vi "Manipulator Intake Handler v3.vi"() -> (14 "Manipulator Mode":T1)   [LabVIEW 2020]
uses:
  Teleop Util/Driver Controls Mode.ctl
  manipulator/Implementation/manipulator Operations.ctl
  dd3cd9fb-53a8-4a5b-9a2b-5e43f9185f3a.vi
  581c7257-3437-4f1d-8e29-cfda183b7fac.vi
  05bd7b36-59a4-46a9-a624-297df426cb22.vi
  <vilib>/Rock Robotics/WPI/Utilities/WPI_GetSetVariantRefNum.vi
  Framework/Robot Global Data.vi
panel:
  in  "Operator Manual Override Scaling":dbl=0.5
  in  "Operator Manual Deadband":dbl=0.2
  in  "Driver Intake Deadband":dbl=0.2 format="%#_13g"
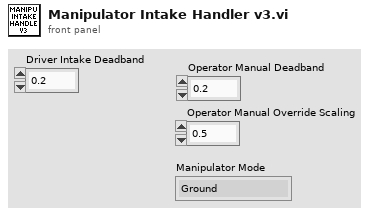
[diagram p1: front panel]
types:
  T1 = typedef "Driver Controls Mode.ctl" = enum16{"Ground", "Scoring"}
  T2 = typedef "manipulator Operations.ctl" = enum16{"Reserve", "Read Current", "Immediate", "Reset Manipulator", "Grid-dy", "Shoot Cubes"}
  T3 = typedef "WPI_JoystickDevRef.ctl" = cluster{"Device":T4}
  T4 = typedef "WPI_JoystickDeviceEnum.ctl" = enum16{"USB 0", "USB 1", "USB 2", "USB 3", "USB 4", "USB 5"}
  T5 = typedef "game object.ctl" = enum16{"Nothing", "Cone", "Cube"}
  T6 = typedef "Cascade Height.ctl" = enum16{"Middle", "High"}
  T7 = typedef "Teleop Manipulator Commands.ctl" = enum16{"idle", "intake cone sideways", "intake cone upright", "intake cone feeder", "intake cube feeder", "intake cube", "score low cone", "score low cube", "score mid cone", "score mid cube", "score high cone", "score high cube", "score mid cone up"}
  T8 = cluster{"Reset Wrist":bool, "Reset Cascade":bool}
  T9 = typedef "Cube Shooting Presets.ctl" = enum16{"shoot low", "shoot mid", "shoot high"}
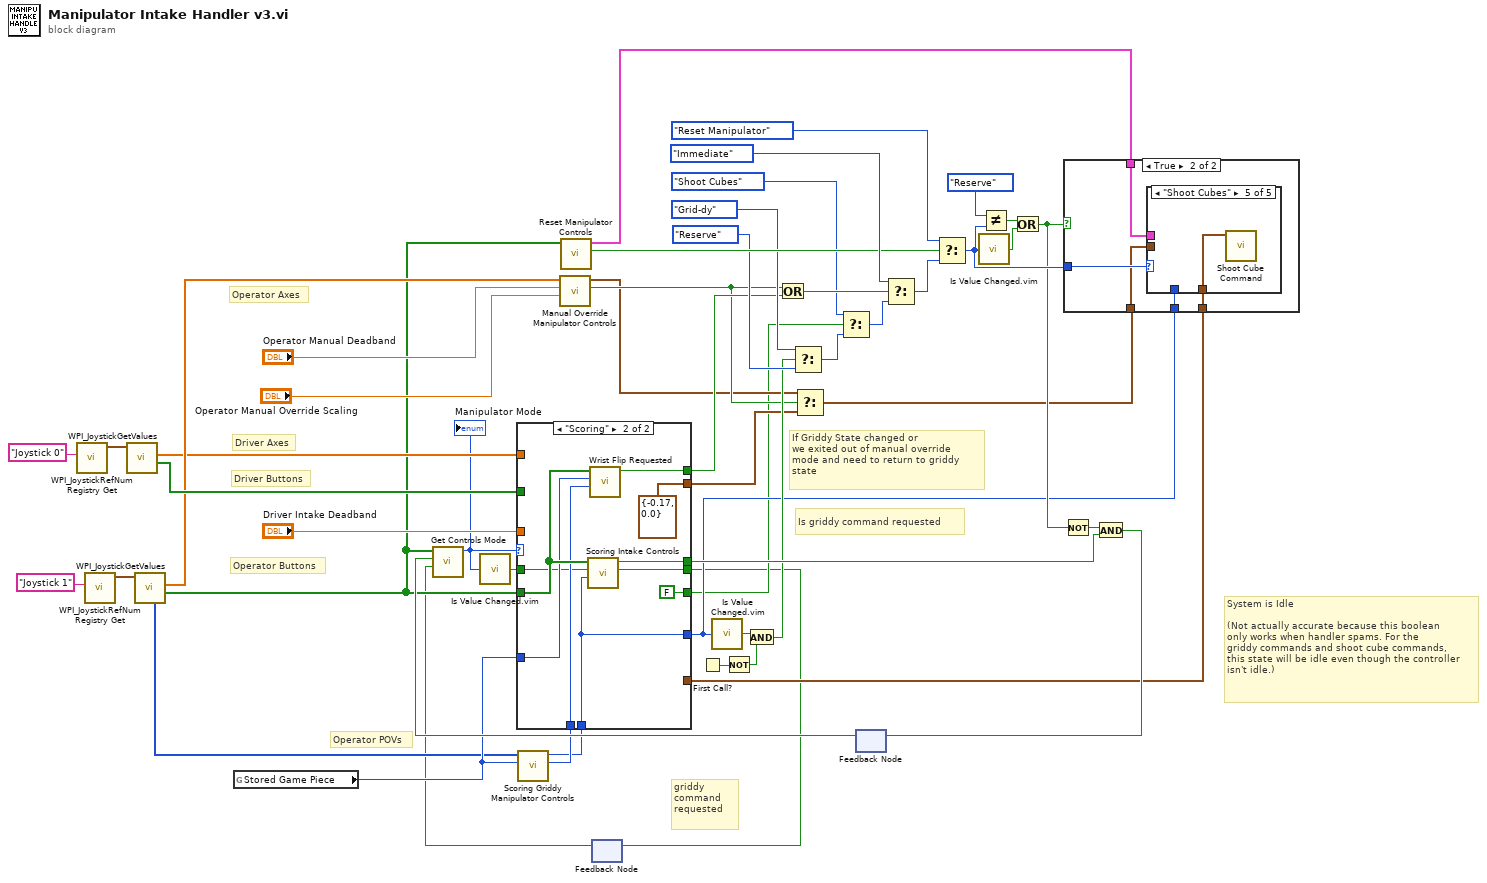
[diagram p0: block diagram]
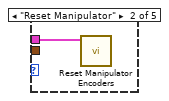
[diagram p4: hidden frame]
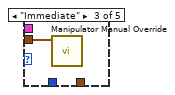
[diagram p5: hidden frame]
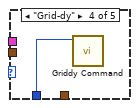
[diagram p6: hidden frame]
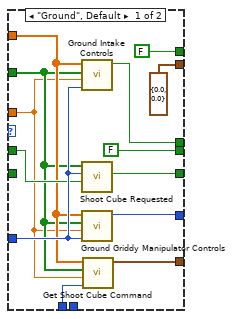
[diagram p7: hidden frame]
diagram:
  # "Operator POVs"
  # "Operator Buttons"
  # "Driver Axes"
  # "Driver Buttons"
  # "Operator Axes"
  # "If Griddy State changed or\nwe exited out of manual override\nmode and need to return to griddy state"
  # "System is Idle\n\n(Not actually accurate because this boolean\nonly works when handler spams. For the\ngriddy commands and shoot cube commands,\nthis state will be idle even though the controller\nisn't idle.)"
  # "griddy command requested"
  # "Is griddy command requested"
  n1 = call <vilib>:"WPI_JoystickRefNum Registry Get.vi"("refnum name"="Joystick 0") -> ("JoystickDevRef"=w18:T3)  [unwired: 1 in, 9 out]
  n2 = call <vilib>:"WPI_JoystickRefNum Registry Get.vi"("refnum name"="Joystick 1") -> ("JoystickDevRef"=w29:T3)  [unwired: 1 in, 9 out]
  n3 = call <vilib>:"WPI_JoystickGetValues.vi"("JoystickDevRef"=w18) -> ("Buttons"=w28:bool[], "Axes"=w26:dbl[])  [unwired: 6 in, 3 out]
  n4 = call <vilib>:"WPI_JoystickGetValues.vi"("JoystickDevRef"=w29) -> ("Buttons"=w25:bool[], "Axes"=w27:dbl[], "POVs"=w24:i16[])  [unwired: 6 in, 2 out]
  n5 = global read "Robot Global Data.vi" "Stored Game Piece"() -> (w32:T5)
  n6 = call "Scoring Griddy Manipulator Controls.vi"("Stored Game Piece"=w32, "Operator POVs"=w24) -> ("Height Preset"=w5:T6, "Griddy Data"=w1:T7)  [unwired: 8 in]
  n7 = call "Manual Override Manipulator Controls.vi"("Manual Override Scaling"="Operator Manual Override Scaling", "Deadband"="Operator Manual Deadband", "Operator Axes"=w27) -> ("Manul Override Requested?"=w15:bool, "Manual Override Data"=w14:cluster{"Wrist Power":dbl, "Cascade Power":dbl})  [unwired: 7 in]
  n8 = call "Reset Manipulator Controls.vi"("Operator Buttons"=w25) -> ("Reset Requested?"=w48:bool, "Reset Parameters"=w41:T8)  [unwired: 9 in]
  n9 = feedback #1() -> (w2:bool)  [unwired: 1 in]
  n10 = First Call?() -> (First Call?: T/F=w22:bool)
  n11 = Not(x=w22) -> (.not. x?=w23:bool)
  n12 = feedback #2() -> (w33:bool)  [unwired: 1 in]
  n13 = call "Get Controls Mode.vi"("Toggle Scoring Mode Requested?"=w2, "System is Idle?"=w33, "Operator Buttons"=w25) -> ("Driver Controls Mode"=w7:T1)  [unwired: 8 in]
  "Manipulator Mode" <- w7
  n14 = call "Is Value Changed.vim"("value"=w7) -> ("changed or first call?"=w6:bool)
  n15 = case shown="\"Scoring\"" w7 {
    tunnel: [w64 w65] -> w19
    tunnel: "Driver Intake Deadband" -> [w54 _]
    tunnel: w26 -> [w56 _]
    tunnel: w28 -> [w55 _]
    tunnel: w25 -> [_ w73]
    tunnel: [w63 w74] -> w36
    tunnel: w32 -> [w60 w71]
    tunnel: [FALSE ("Wrist Flip Requested?") w72] -> w16
    tunnel: [cluster{"Wrist Power":dbl, "Cascade Power":dbl} {"Wrist Power"=0.0, "Cascade Power"=0.0} ("Wrist Flip Power") cluster{"Wrist Power":dbl, "Cascade Power":dbl} {"Wrist Power"=-0.17, "Cascade Power"=0.0} ("Wrist Flip Power")] -> w12
    tunnel: w5 -> [w57 w70]
    tunnel: [w59 FALSE ("Shoot Cube Requested?")] -> w8
    tunnel: w6 -> [w58 w67]
    tunnel: [w53 _] -> w4
    tunnel: [FALSE ("Lower Cascade?") w66] -> w3
    tunnel: w1 -> [_ w65]
    frame "Ground", Default {
      n16 = call "Ground Intake Controls.vi"("Stored Game Piece"=w60, "Deadband"=w54, "Driver Buttons"=w55, "Driver Axes"=w56) -> ("Is Idle?"=w63:bool)  [unwired: 7 in]
      n17 = call "Shoot Cube Requested.vi"("Other Command Requested?"=w58, "Stored Game Piece"=w60, "Driver Buttons"=w55) -> ("Shoot Cube Pressed?"=w59:bool)  [unwired: 7 in, 1 out]
      n18 = call "Ground Griddy Manipulator Controls.vi"("Stored Game Piece"=w60, "Deadband"=w54, "Driver Buttons"=w55, "Driver Axes"=w56) -> ("Ground Griddy Manipulator Controls"=w64:T7)  [unwired: 7 in]
      n19 = call "Get Shoot Cube Command.vi"("Height Preset"=w57, "Deadband"=w54, "Driver Buttons"=w55, "Driver Axes"=w56) -> ("Shoot Cube Preset"=w53:cluster{"Shot Preset":T9})  [unwired: 7 in]
    }
    frame "Scoring" {
      n20 = call "Scoring Intake Controls.vi"("Griddy Data"=w65, "Reset?"=w67, "Operator Buttons"=w73) -> ("Lower Cascade?"=w66:bool, "Is Idle?"=w74:bool)  [unwired: 7 in]
      n21 = call "Wrist Flip Requested.vi"("Height Preset"=w70, "Stored Game Piece"=w71, "Operator Buttons"=w73) -> ("Wrist Flip Requested?"=w72:bool)  [unwired: 8 in]
    }
  }
  n22 = feedback-in #1(w3) -> ()
  n23 = call "Is Value Changed.vim"("value"=w19) -> ("changed or first call?"=w21:bool)
  n24 = And(x=w21, y=w23) -> (x .and. y?=w20:bool)
  n25 = Or(x=w15, y=w16) -> (x .or. y?=w17:bool)
  n26 = Select(t=manipulator_Operations."Grid-dy" ("Operation"), s=w20, f=manipulator_Operations."Reserve" ("Operation")) -> (s? t:f=w10:T2)
  n27 = Select(t=w14, s=w15, f=w12) -> (s? t:f=w13:cluster{"Wrist Power":dbl, "Cascade Power":dbl})
  n28 = Select(t=manipulator_Operations."Shoot Cubes" ("Operation"), s=w8, f=w10) -> (s? t:f=w11:T2)
  n29 = Select(t=manipulator_Operations."Immediate" ("Operation"), s=w17, f=w11) -> (s? t:f=w49:T2)
  n30 = Select(t=manipulator_Operations."Reset Manipulator" ("Operation"), s=w48, f=w49) -> (s? t:f=w42:T2)
  n31 = call "Is Value Changed.vim"("value"=w42) -> ("changed or first call?"=w45:bool)
  n32 = Not Equal?(x=manipulator_Operations."Reserve", y=w42) -> (x != y?=w44:bool)
  n33 = Or(x=w44, y=w45) -> (x .or. y?=w38:bool)
  n34 = Not(x=w38) -> (.not. x?=w37:bool)
  n35 = case shown="True" w38 {
    tunnel: w42 -> [_ w79]
    tunnel: w19 -> [_ w78]
    tunnel: w41 -> [_ w77]
    tunnel: w13 -> [_ w76]
    tunnel: w4 -> [_ w75]
    frame False {
    }
    frame True {
      n36 = case shown="\"Shoot Cubes\"" w79 {
        tunnel: w78 -> [_ _ _ w82 _]
        tunnel: w77 -> [_ w80 _ _ _]
        tunnel: w76 -> [_ _ w81 _ _]
        tunnel: w75 -> [_ _ _ _ w83]
        frame Default {
        }
        frame "Reset Manipulator" {
          n37 = call "Reset Manipulator Encoders.vi"("Reset Parameters"=w80) -> ()  [unwired: 10 in, 1 out]
        }
        frame "Immediate" {
          n38 = call "Manipulator Manual Override.vi"("Immediate Parameters"=w81) -> ()  [unwired: 10 in, 1 out]
        }
        frame "Grid-dy" {
          n39 = call "Griddy Command.vi"("Griddy Command"=w82) -> ()  [unwired: 10 in, 1 out]
        }
        frame "Shoot Cubes" {
          n40 = call "Shoot Cube Command.vi"("Shoot Cube Parameters"=w83) -> ()  [unwired: 10 in, 1 out]
        }
      }
    }
  }
  n41 = And(x=w37, y=w36) -> (x .and. y?=w35:bool)
  n42 = feedback-in #2(w35) -> ()
